vi "SV Compute Statistical Level from Histogram.vi"(0 "histogram":cluster{"bin centers":dbl[], "counts":u64[]}(graph), 5 "range (-10..10)":cluster{"minimum":dbl, "maximum":dbl}={"minimum"=-10.0, "maximum"=10.0}, 7 "histogram counts":T1, 9 "N (50 %)":dbl=50.0 min=0.0 max=100.0 step=0.5) -> (4 "cumulative count":cluster{"bin centers":dbl[], "count":u64[]}(graph), 6 "L_N":dbl min=0.0 max=100.0 step=0.5 format="%_4g")   [LabVIEW 2017]
doc: "Use this VI to return <B>L_N</B> levels where L_N is the level which N % of the values exceed. For example, L50 represents the median, where 50 % of the values are greater than L_N and 50 % are lower. L90 is commonly used as a noise baseline, as 90 % of the values exceed L_N. L10 is commonly used as a measure of peak levels because it corresponds to the highest 10 % of levels."
uses:
  <vilib>/addons/_NISVFA/_Shared subVIs/Controls/svc_Histogram Counts.ctl
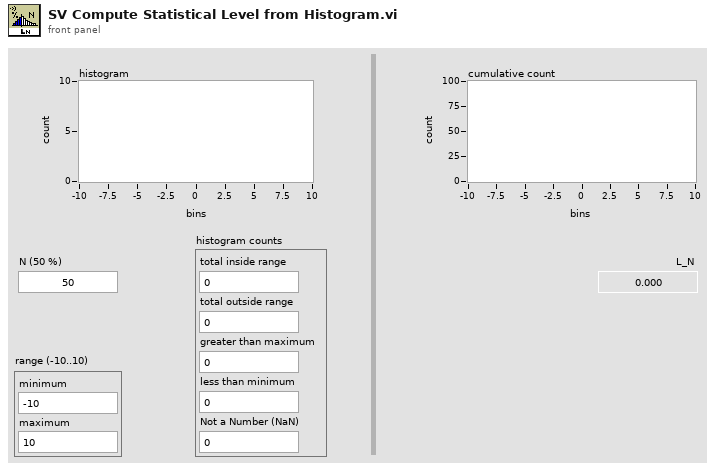
[diagram p1: front panel]
types:
  T1 = typedef "svc_Histogram Counts.ctl" = cluster{"total inside range":u64, "total outside range":u64, "greater than maximum":u64, "less than minimum":u64, "Not a Number (NaN)":u64}
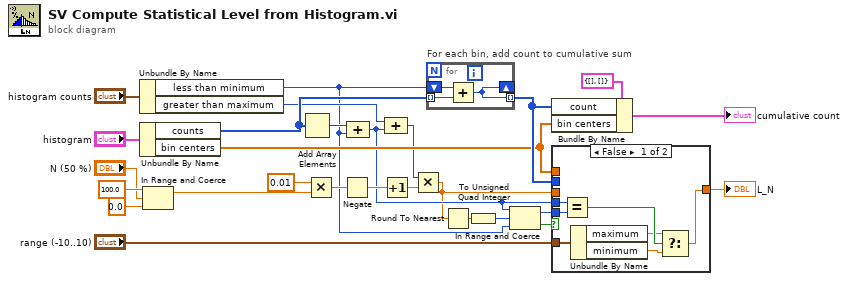
[diagram p0: block diagram]
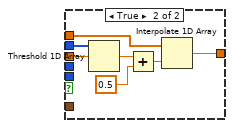
[diagram p2: hidden frame]
diagram:
  n1 = Unbundle By Name("histogram counts") -> ("less than minimum"=w2:u64, "greater than maximum"=w7:u64)
  n2 = Unbundle By Name("histogram") -> ("counts"=w23:u64[], "bin centers"=w18:dbl[])
  n3 = In Range and Coerce(upper limit=100.0, x="N (50 %)", lower limit=0.0) -> (coerced(x)=w3:dbl)  [unwired: 1 out]
  n4 = Add Array Elements(numeric array=w23) -> (sum=w22:u64)
  n5 = Multiply(x=0.01, y=w3) -> (x*y=w19:dbl)
  n6 = Negate(x=w19) -> (-x=w17:dbl)
  n7 = Compound Arithmetic op=ADD(w22, w2) -> (w10:u64)
  n8 = Increment(x=w17) -> (x+1=w16:dbl)
  n9 = Compound Arithmetic op=ADD(w7, w10) -> (w15:u64)
  n10 = Multiply(x=w15, y=w16) -> (x*y=w1:dbl)
  n11 = for "For each bin, add count to cumulative sum" {
    shift-right: [w28] -> _
    shift-left: w2 -> [w30]
    tunnel: w23 -> [w29] mode=indexing
    tunnel: [w28] -> w21 mode=indexing
    n12 = Add(x=w30, y=w29) -> (x+y=w28:u64)
  }
  n13 = Round To Nearest(number=w1) -> (nearest integer value=w13:dbl)
  n14 = To Unsigned Quad Integer(1:w13) -> (0:w14:u64)
  n15 = In Range and Coerce(upper limit=w10, x=w14, lower limit=w2) -> (coerced(x)=w11:u64, In Range?=w12:bool)
  n16 = Bundle By Name(cluster=cluster{"bin centers":dbl[], "count":u64[]} {"bin centers"=[], "count"=[]} ("Cluster 2"), "count"=w21, "bin centers"=w18) -> (→"cumulative count":cluster{"bin centers":dbl[], "count":u64[]})
  n17 = case shown="False" w12 {
    tunnel: w21 -> [_ w44]
    tunnel: w18 -> [_ w42]
    tunnel: w1 -> [_ w38]
    tunnel: w11 -> [w37 _]
    tunnel: w10 -> [w36 _]
    tunnel: [w34 w41] -> w9
    tunnel: "range (-10..10)" -> [w33 _]
    frame False {
      n18 = Equal?(x=w36, y=w37) -> (x = y?=w35:bool)
      n19 = Unbundle By Name(w33) -> ("maximum"=w32:dbl, "minimum"=w31:dbl)
      n20 = Select(t=w32, s=w35, f=w31) -> (s? t:f=w34:dbl)
    }
    frame True {
      n21 = Threshold 1D Array(2:w38, 3:w44) -> (0:w43:dbl)  [unwired: 1 in]
      n22 = Add(x=w43, y=0.5) -> (x+y=w39:dbl)
      n23 = Interpolate 1D Array(1:w39, 2:w42) -> (0:w41:dbl)
    }
  }
  "L_N" <- w9
